vi "getEventErrorCode.vi"(8 "error in (no error)":errorcluster, 11 "SALCommunicatorView in":refnum<class "SALCommunicatorView.lvclass">) -> (0 "error out":errorcluster, 3 "SALCommunicatorView out":refnum<class "SALCommunicatorView.lvclass">)   [LabVIEW 2016, in "SALCommunicatorView.lvclass"]
uses:
  SALCommunicatorView.lvclass
  ts_sallv_exa/DataTypes/logevent_ErrorCode.ctl
  ts_sallv_exa/SALLV_EXA.lvlib
panel:
  out "logevent_ErrorCode_Ctl out":T1
  out "function return":i32
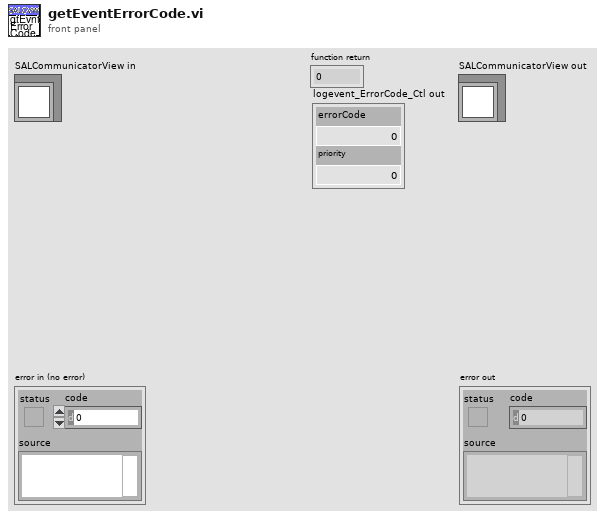
[diagram p1: front panel]
types:
  T1 = typedef "SALLV_EXA.lvlib/logevent_ErrorCode.ctl" = cluster{"errorCode":i32, "priority":i32}
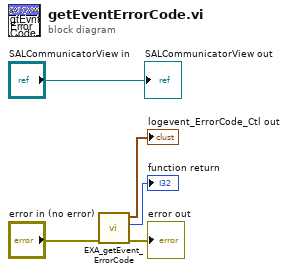
[diagram p0: block diagram]
diagram:
  n1 = call "EXA_getEvent_ErrorCode.vi"("error in (no error)"="error in (no error)") -> ("error out"=→"error out":errorcluster, "function return"=→"function return":i32, "logevent_ErrorCode_Ctl out"=→"logevent_ErrorCode_Ctl out":T1)  [unwired: 8 in]
  "SALCommunicatorView out" <- "SALCommunicatorView in"
